vi "pySSHInterface.vi"(6 "Task":enum16{"Init", "Read", "Write", "Close"}(ring), 10 "String to write":string, 11 "IP Address":string) -> (2 "reply":string)   [LabVIEW 2016]
uses:
  <vilib>/httpClient/LabVIEWHTTPClient.lvlib
  <vilib>/httpClient/POSTBuffer.vi
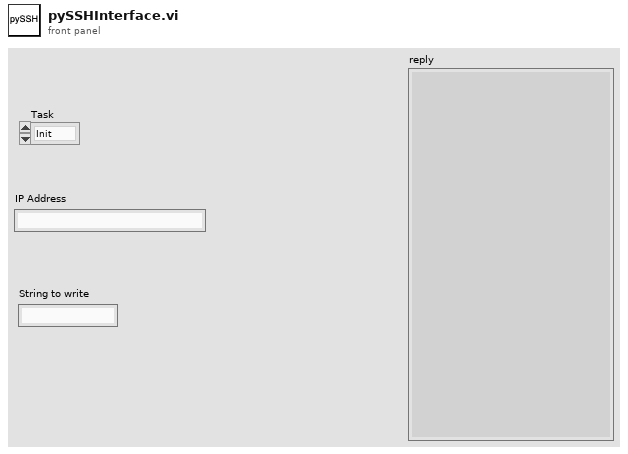
[diagram p1: front panel]
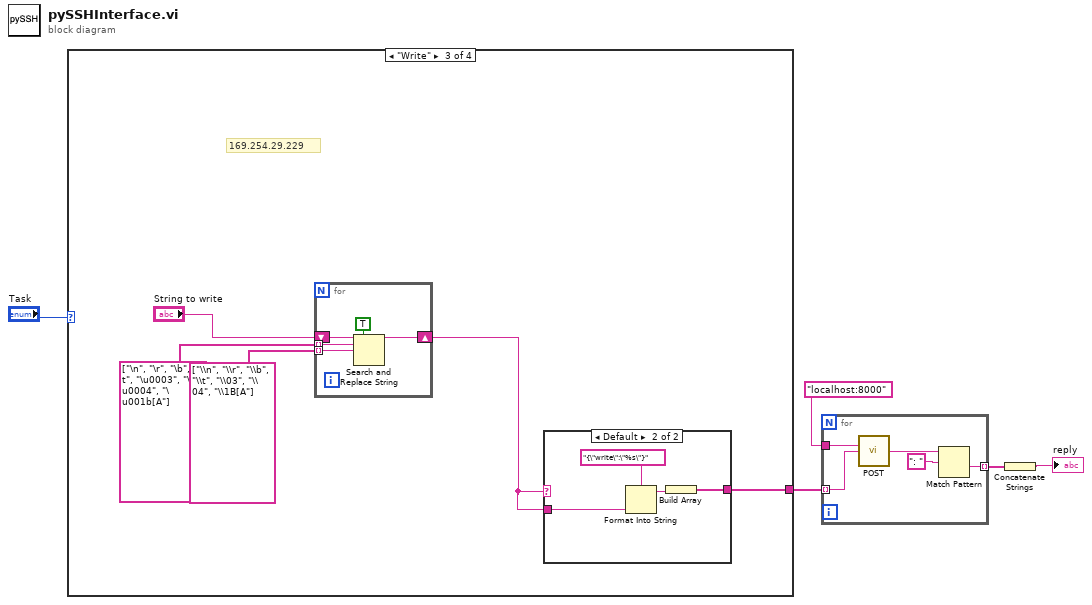
[diagram p0: block diagram]
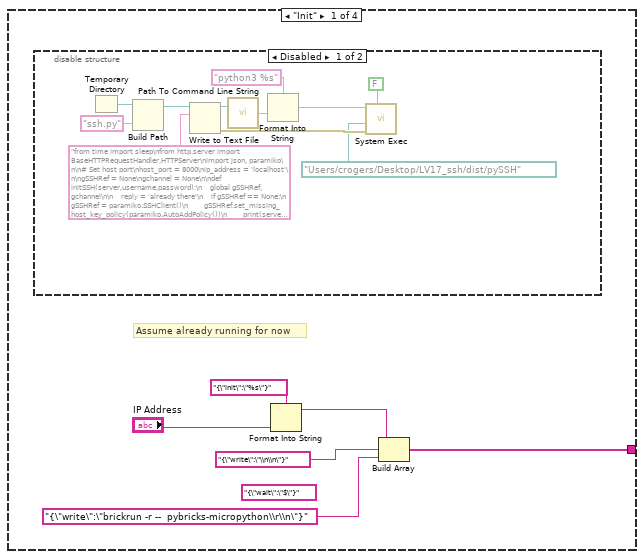
[diagram p2: hidden frame]
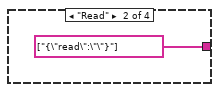
[diagram p4: hidden frame]
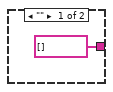
[diagram p5: hidden frame]
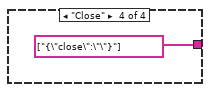
[diagram p6: hidden frame]
diagram:
  n1 = case shown="\"Write\"" "Task" {
    tunnel: [w7 string[] ["{\"read\":\"\"}"] ("Array") w27 string[] ["{\"close\":\"\"}"] ("Array")] -> w2
    frame "Init" {
      (unwired) "{\"wait\":\"$\"}" ("buffer")
      # "Assume already running for now"
      n2 = disable-structure shown="Disabled" {
        frame Disabled {
          n3 = Temporary Directory() -> (w21:path)
          n4 = Build Path(base path=w21, name or relative path="ssh.py") -> (appended path=w16:path)
          n5 = Write to Text File(file (use dialog)=w16, text="from time import sleep\nfrom http.server import BaseHTTPRequestHandler,HTTPServer\nimport json, paramiko\n\n# Set host port\nhost_port = 8000\nip_address = 'localhost'\n\ngSSHRef = None\ngchannel = None\n\ndef initSSH(server,username,password):\n    global gSSHRef, gchannel\n\n    reply = 'already there'\n    if gSSHRef == None:\n        gSSHRef = paramiko.SSHClient()\n        gSSHRef.set_missing_host_key_policy(paramiko.AutoAddPolicy())\n        print(server + username + password)\n        result = gSSHRef.connect(server, username=username, password=password, timeout = 5)\n        reply = str(result)\n        gchannel = gSSHRef.invoke_shell()\n        gchannel.settimeout(0)\n    return reply\n\ndef closeSSH():\n    global gSSHRef, gchannel\n    if gchannel != None:\n        gchannel.close()\n    if gSSHRef != None:\n        gSSHRef.close()\n    gSSHRef = None\n    gchannel = None\n    return True\n\ndef writeSSH(string):\n    reply = 'no reference'\n    if gSSHRef != None:\n        reply = 'no file'\n        if gchannel != None:\n            size = gchannel.send(string.encode())\n            reply = str(size)\n    return reply\n\ndef readSSH():\n    reply = 'no reference'\n    if gSSHRef != None:\n        reply = 'no file'\n        if gchannel != None:\n            reply = ''\n            if gchannel.recv_ready():\n                reply = gchannel.recv(9999).decode()\n\n    return(reply)\n\nclass MyServer(BaseHTTPRequestHandler):\n\n    def do_HEAD(self):\n        self.send_response(200)\n        self.send_header('Content-type', 'text/html')\n        self.end_headers()\n\n    def _redirect(self, path):\n        self.send_response(303)\n        self.send_header('Content-type', 'text/html')\n        self.send_header('Location', path)\n        self.end_headers()\n\n    def do_GET(self):\n\n        self.do_HEAD()\n\n    def do_POST(self):\n\n        content_length = int(self.headers['Content-Length'])  # Get the size of data\n        post_data = self.rfile.read(content_length).decode('utf-8')  # Get the data\n        print(post_data)\n        data_array = json.loads(post_data)\n        print(data_array)\n        for data in data_array:\n            print(data)\n            if 'test' in data:\n                print(data['test'])\n                pageContent = 'got: ' + data['test']\n            elif 'init' in data:\n                server = data['init']\n                pageContent = 'init: ' + str(initSSH(server,\"robot\",\"maker\"))\n            elif 'write' in data:\n                pageContent = 'wrote: ' + writeSSH(data['write'])\n            elif 'wait' in data:\n                reply = ''\n                while not data['wait'] in reply:\n                    sleep(1)\n                    reply = reply + readSSH()\n                    print(reply)\n                pageContent = 'wait: ' + reply\n            elif 'read' in data:\n                pageContent = 'read: ' + readSSH()\n            elif 'close' in data:\n                success = closeSSH()\n                pageContent = 'closed' if success else 'failed to close'\n            else:\n                pageCommand = 'Not Supported Command'\n\n        self.wfile.write(pageContent.encode(\"utf-8\"))\n       \n\n# Create Webserver\nif __name__ == '__main__':\n\n    http_server = HTTPServer((ip_address, host_port),MyServer)\n    print(\"Server Starts - %s:%s\" % (ip_address, host_port))\n\n    try:\n        http_server.serve_forever()\n    except KeyboardInterrupt:\n        http_server.server_close()\n        print(\"\\n-------------------EXIT-------------------\")\n\n\n'''\nclass MySSH():\n    def __init(server,username,password):\n        self.server = server\n        self.username = username\n        self.password = password\n        self.gSSHRef = None\n        gchannel = None\n    def init():\n        reply = 'already there'\n        if self.gSSHRef == None:\n            self.gSSHRef = paramiko.SSHClient()\n            self.gSSHRef.set_missing_host_key_policy(paramiko.AutoAddPolicy())\n            result = self.gSSHRef.connect(self.server, self.username, self.password, timeout = 5)\n            reply = str(result)\n            gchannel = self.gSSHRef.invoke_shell()\n            gchannel.settimeout(0)\n        return reply\n    def close():\n        if gchannel != None:\n            gchannel.close()\n        if gSSHRef != None:\n            gSSHRef.close()\n        return True\n    def write(string):\n        reply = 'no reference'\n        if gSSHRef != None:\n            reply = 'no file'\n        if gchannel != None:\n            size = gchannel.send(string.encode())\n            reply = str(size)\n        return reply\n    def read()\n        reply = 'no reference'\n        if gSSHRef != None:\n            reply = 'no file'\n            if gchannel != None:\n                reply = ''\n                if gchannel.recv_ready():\n                    reply = gchannel.recv(9999).decode()\n\n        return(reply)\n        '''\n" ("buffer")) -> (error out=w18:errorcluster)  [unwired: 2 in, 2 out]
          n6 = call <vilib>:"Path To Command Line String.vi"("path"=w16) -> ("string"=w15:string)
          n7 = Format Into String(format string="python3 %s" ("command line"), w15) -> (resulting string=w14:string)  [unwired: 2 in, 1 out]
          n8 = call <vilib>:"System Exec.vi"("wait until completion? (T)"=FALSE, "error in (no error)"=w18, "working directory"=path "/Users/crogers/Desktop/LV17_ssh/dist/pySSH", "command line"=w14) -> ()  [unwired: 4 in, 4 out]
        }
        frame Enabled {
        }
      }
      n9 = Format Into String(format string="{\"init\":\"%s\"}" ("buffer"), "IP Address") -> (resulting string=w9:string)  [unwired: 2 in, 1 out]
      n10 = Build Array(w9, "{\"write\":\"\\n\\n\"}" ("buffer"), "{\"write\":\"brickrun -r --  pybricks-micropython\\r\\n\"}" ("buffer")) -> (w7:string[])
    }
    frame "Read" {
    }
    frame "Write" {
      # "169.254.29.229"
      n11 = for {
        tunnel: string[] ["\n", "\r", "\b", "\t", "\u0003", "\u0004", "\u001b[A"] -> [w29] mode=indexing
        tunnel: string[] ["\\n", "\\r", "\\b", "\\t", "\\03", "\\04", "\\1B[A"] -> [w28] mode=indexing
        shift-right: [w31] -> w23
        shift-left: "String to write" -> [w30]
        n12 = Search and Replace String(replace all?=TRUE ("replace all? (F)"), input string=w30, search string=w29, replace string=w28) -> (result string=w31:string)  [unwired: 4 in, 3 out]
      }
      n13 = case shown="Default" w23 {
        tunnel: w23 -> [_ w37]
        tunnel: [string[] [] w34] -> w27
        frame "" {
        }
        frame Default {
          n14 = Format Into String(format string="{\"write\":\"%s\"}" ("buffer"), w37) -> (resulting string=w35:string)  [unwired: 2 in, 1 out]
          n15 = Build Array(w35) -> (w34:string[])
        }
      }
    }
    frame "Close" {
    }
  }
  n16 = for {
    tunnel: "localhost:8000" ("url") -> [w43]
    tunnel: w2 -> [w42] mode=indexing
    tunnel: [w39] -> w4 mode=indexing
    n17 = call-poly <vilib>:"POST.vi"("url"=w43, "buffer"=w42) -> ("body"=w40:string)  [unwired: 10 in, 3 out]
    n18 = Match Pattern(string=w40, regular expression=": ") -> (after substring=w39:string)  [unwired: 1 in, 3 out]
  }
  n19 = Concatenate Strings(w4) -> (→"reply":string)
